vi "Pseudo Wigner-Ville Distribution.vi"() -> ()   [LabVIEW 2023]
doc: "This example shows how to use the TFA Cohen VI to compute the Pseudo Wigner-Ville Distribution (PWVD).\n\n<b>Instructions</b>:\n1) Run this VI and observe the <b>Pseudo Wigner-Ville Distribution</b>.\n2) Change the value of <b>Alpha</b> and observe the cross-term interference. Increase <b>Alpha</b> and notice the cross-term interference fade away. Increasing <b>Alpha</b> causes the time-frequency resolution to deteriorate. Decreasing <b>Alpha</b> enhances the time-frequency resolution. As <b>Alpha</b> approaches zero, the distribution converges to the Wigner-Ville Distribution (WVD).\n3) Browse the Block Diagram to learn how to implement the PWVD by using the TFA Cohen VI."
uses:
  <vilib>/addons/Time Frequency Analysis/Spectrogram.llb/TFA Cohen (Waveform).vi
  <vilib>/addons/Time Frequency Analysis/_control.llb/TFA Configure Spectrogram Indicator (Predefined Color Table).vi
  <vilib>/addons/_Advanced Signal Processing/NI_AdvSigProcTFA.lvlib
panel:
  in  "Alpha":dbl=0.001 min=0.0 step=0.001 format="%.3f"
  in  "Data":u16(ring) items=["PC Fan"=0, "Noisy Chirps"=1, "TDR 1"=2, "TDR 2"=3, "Liquefaction"=4, "Liquefaction Free"=5, "Aneurysm"=6, "Bat"=7, "RF"=8, "Two Gaussian"=9, "Three Gaussian"=10, "Chirp"=11, "Gaussian Chirp"=12, "Cross Chirp"=13, "Doppler"=14, "HOP"=15, "TF Sine"=16, "Three Tone"=17, "Four Tone"=23, "Blood Flow Doppler (phase a)"=20, "Blood Flow Doppler (phase b)"=21, "Heart sound"=22, "Random Noise"=19]
  in  "Stop":bool
  out "aspt-left-top":bool
  out "Pseudo Wigner-Ville Distribution":dbl[][](graph)
  out "Source Signal":waveform(dbl)(graph)
  # "Overview: Shows how to use the TFA Cohen VI to compute the Pseudo Wigner-Ville Distribution (PWVD).\nRequirements: LabVIEW Full Development System, Advanced Signal Processing Toolkit\nInstructions: \n1. Run this VI and observe the Pseudo Wigner-Ville Distribution.\n2. Change the value of Alpha and observe the cross-term interference. Increase Alpha and notice the cross-term interference fade away. Increasing Alpha causes the time-frequency resolution to deteriorate. Decreasing Alpha enhances the time-frequency resolution. As Alpha approaches zero, the distribution converges to the Wigner-Ville Distribution (WVD).\n3. Browse the Block Diagram to learn how to implement the PWVD by using the TFA Cohen VI.\n4. Click Stop to stop the VI."
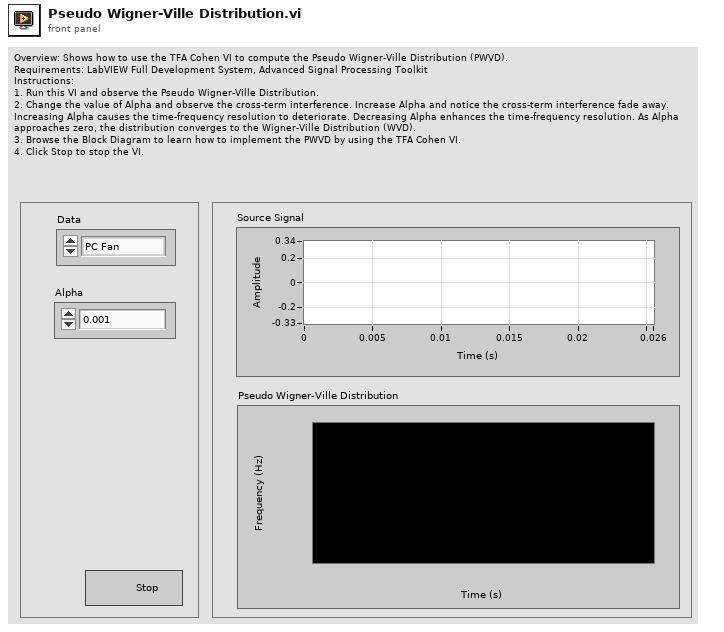
[diagram p1: front panel]
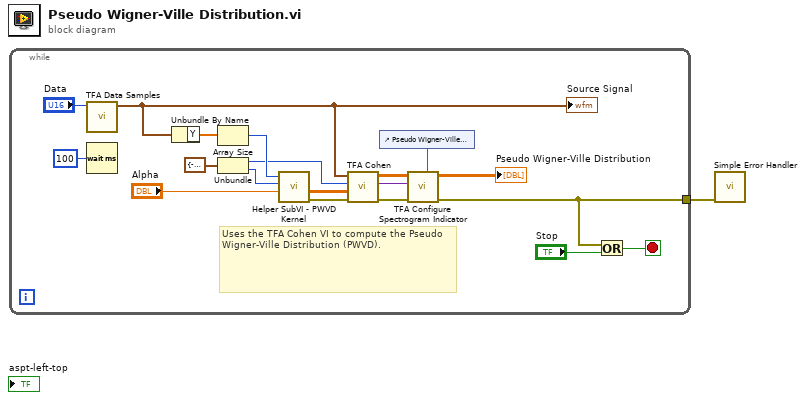
[diagram p0: block diagram]
diagram:
  n1 = while {
    tunnel: [w2] -> w1
    stop <- w3 stop-if-true
    # "Uses the TFA Cohen VI to compute the Pseudo Wigner-Ville Distribution (PWVD)."
    n2 = call <vilib>:"TFA Data Samples.vi"("data"="Data") -> ("signal"=w8:waveform(dbl))  [unwired: 10 out]
    "Source Signal" <- w8
    n3 = Wait (ms)(milliseconds to wait=u32 100 ("millisecond multiple")) -> ()  [unwired: 1 out]
    n4 = Unbundle By Name(w8) -> ("Y"=w12:dbl[])
    n5 = Array Size(array=w12) -> (size(s)=w13:i32)
    n6 = Unbundle(cluster{"time steps":i32, "frequency bins":i32} {"time steps"=-1, "frequency bins"=512} ("time-frequency sampling info")) -> ("time steps"=w10:i32, "frequency bins"=w9:i32)
    n7 = call "Helper SubVI - PWVD Kernel.vi"("alpha"="Alpha", "num of frequency bins"=w9, "length"=w13) -> ("error out"=w14:errorcluster, "kernel"=w11:dbl[][])  [unwired: 7 in]
    n8 = call-poly <vilib>:"TFA Cohen.vi"("error in (no error)"=w14, "kernel"=w11, "time steps"=w10, "signal"=w8) -> ("error out"=w6:errorcluster, "scale info"=w5:variant, "spectrogram"=w7:dbl[][])  [unwired: 5 out]
    n9 = control-ref of="Pseudo Wigner-Ville Distribution"() -> (w18:refnum<vi>)
    n10 = call-poly <vilib>:"TFA Configure Spectrogram Indicator.vi"("reference of TF spectrogram indicator"=w18, "error in (no error)"=w6, "scale info"=w5, "spectrogram"=w7) -> ("error out"=w2:errorcluster, "TF spectrogram indicator"=→"Pseudo Wigner-Ville Distribution":dbl[][])  [unwired: 3 in, 3 out]
    n11 = Or(x=w2, y="Stop") -> (x .or. y?=w3:bool)
  }
  n12 = call <vilib>:"Simple Error Handler.vi"("error in (no error)"=w1) -> ()  [unwired: 4 in, 5 out]
